vi "resize_table_columns.vi"(7 "vi_reference":refnum<vi>, 8 "error in (no error)":errorcluster, 10 "configuration":T1=enum."all", 11 "listbox_reference":refnum<vi>) -> (0 "error out":errorcluster)   [LabVIEW 2015, in "lv-pagination.lvlib"]
doc: "This VI can be used to automatically determine the appropriate value for column width and row height depending on the contents of the cells themselves."
uses:
  lv-pagination.lvlib
  _controls/configuratin_resize.ctl
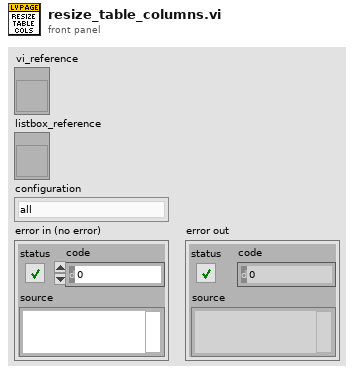
[diagram p1: front panel]
types:
  T1 = typedef "lv-pagination.lvlib/configuratin_resize.ctl" = enum16{"<resize_config>", "header", "contents", "all", "best_fit"}
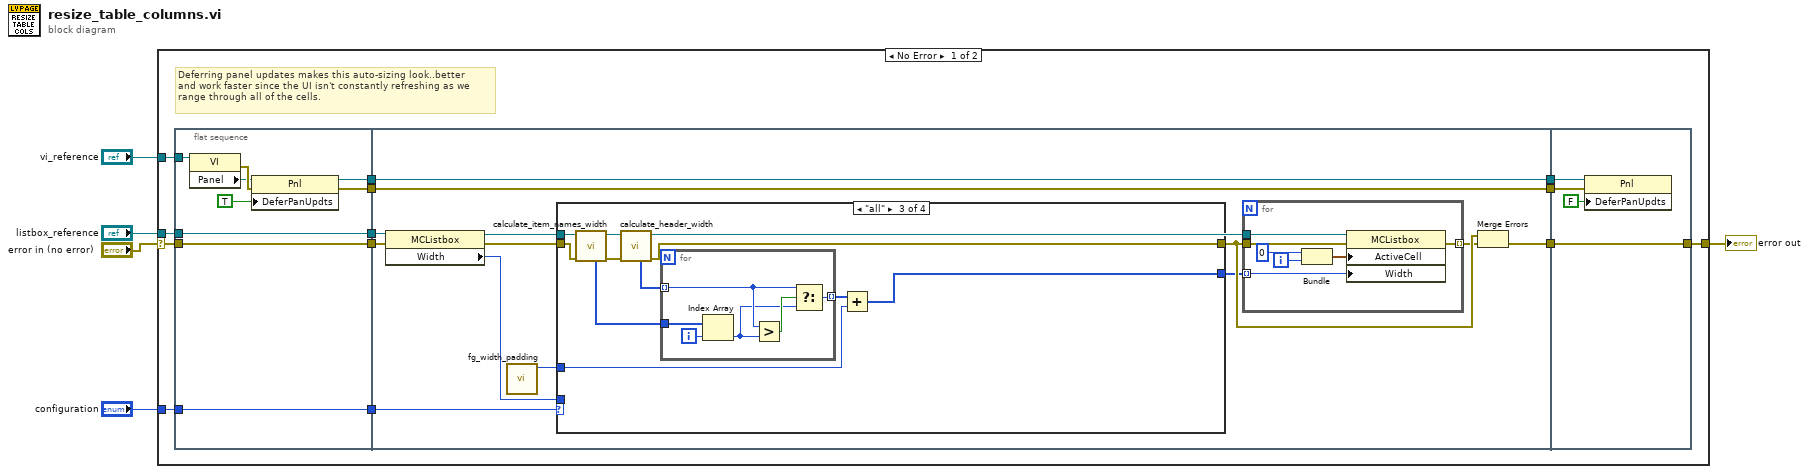
[diagram p0: block diagram]
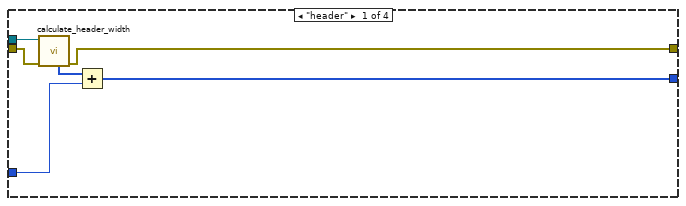
[diagram p2: hidden frame]
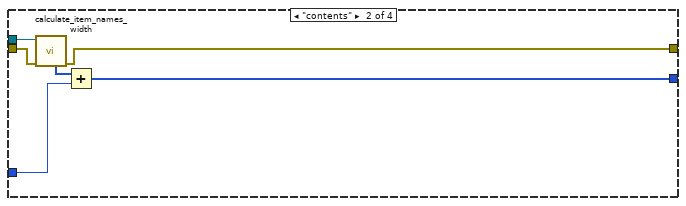
[diagram p3: hidden frame]
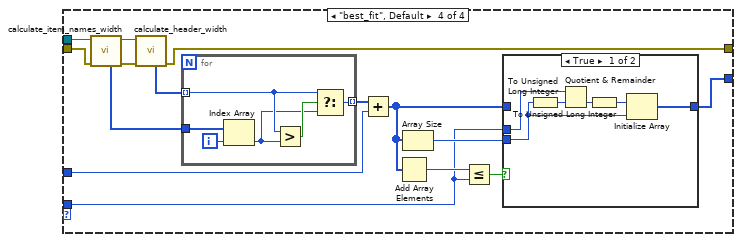
[diagram p4: hidden frame]
diagram:
  n1 = case shown="No Error" "error in (no error)" {
    selector: "error in (no error)" -> [w6 w106]
    tunnel: "configuration" -> [w10 _]
    tunnel: "listbox_reference" -> [w9 _]
    tunnel: [w8 w106] -> w3
    tunnel: "vi_reference" -> [w7 _]
    frame No Error {
      # "Deferring panel updates makes this auto-sizing look..better\nand work faster since the UI isn't constantly refreshing as we\nrange through all of the cells."
      n2 = flat-sequence {
        tunnel: w9 -> [w26]
        tunnel: w10 -> [w27]
        tunnel: [w27] -> w18
        tunnel: [w26] -> w17
        tunnel: w7 -> [w22]
        tunnel: [w21] -> w16
        tunnel: [w20] -> w15
        tunnel: [w19] -> w14
        tunnel: w6 -> [w19]
        tunnel: w18 -> [w40]
        tunnel: w17 -> [w39]
        tunnel: [w38] -> w13
        tunnel: w16 -> [w29]
        tunnel: w15 -> [w30]
        tunnel: [w30] -> w12
        tunnel: [w29] -> w11
        tunnel: w14 -> [w28]
        tunnel: [w105] -> w8
        tunnel: w13 -> [w105]
        tunnel: w12 -> [w104]
        tunnel: w11 -> [w103]
        frame #0 {
          n3 = property class="VI"(reference=w22) -> (error out=w25:errorcluster, "Panel"=w23:refnum<vi>)  [unwired: 1 in, 1 out]
          n4 = property class="Pnl"(reference=w23, error in=w25, "DeferPanUpdts"=TRUE) -> (reference out=w20:refnum<vi>, error out=w21:errorcluster)
        }
        frame #1 {
          n5 = property on="Property Node" class="MCListbox"(reference=w39, error in=w28) -> (reference out=w32:refnum<vi>, error out=w34:errorcluster, "Width"=w33:u32)
          n6 = call "fg_width_padding.vi"() -> ("width_padding out"=w31:u32)  [unwired: 10 in, 1 out]
          n7 = case shown="\"all\"" w40 {
            tunnel: [w46 w51 w55 w71] -> w35
            tunnel: w33 -> [_ _ _ w69]
            tunnel: w31 -> [w45 w52 w56 w76]
            tunnel: w32 -> [w44 w50 w53 w68]
            tunnel: w34 -> [w43 w49 w61 w81]
            tunnel: [w41 w47 w54 w75] -> w37
            frame "header" {
              n8 = call "calculate_header_width.vi"("error in (no error)"=w43, "listbox_reference"=w44) -> ("error out"=w41:errorcluster, "width []"=w42:u32[])  [unwired: 7 in, 1 out]
              n9 = Add(x=w42, y=w45) -> (x+y=w46:u32[])
            }
            frame "contents" {
              n10 = call "calculate_item_names_width.vi"("error in (no error)"=w49, "listbox_reference"=w50) -> ("error out"=w47:errorcluster, "width []"=w48:u32[])  [unwired: 7 in, 1 out]
              n11 = Add(x=w48, y=w52) -> (x+y=w51:u32[])
            }
            frame "all" {
              n12 = call "calculate_item_names_width.vi"("error in (no error)"=w61, "listbox_reference"=w53) -> ("error out"=w60:errorcluster, "width []"=w58:u32[])  [unwired: 7 in, 1 out]
              n13 = call "calculate_header_width.vi"("error in (no error)"=w60, "listbox_reference"=w53) -> ("error out"=w54:errorcluster, "width []"=w59:u32[])  [unwired: 7 in, 1 out]
              n14 = for {
                tunnel: w59 -> [w64] mode=indexing
                tunnel: w58 -> [w67]
                tunnel: [w62] -> w57 mode=indexing
                i -> [w66]
                n15 = Index Array(array=w67, index=w66) -> (element=w63:u32)
                n16 = Greater?(x=w64, y=w63) -> (0:w65:bool)
                n17 = Select(t=w64, s=w65, f=w63) -> (s? t:f=w62:u32)
              }
              n18 = Add(x=w57, y=w56) -> (x+y=w55:u32[])
            }
            frame "best_fit", Default {
              n19 = call "calculate_item_names_width.vi"("error in (no error)"=w81, "listbox_reference"=w68) -> ("error out"=w80:errorcluster, "width []"=w78:u32[])  [unwired: 7 in, 1 out]
              n20 = call "calculate_header_width.vi"("error in (no error)"=w80, "listbox_reference"=w68) -> ("error out"=w75:errorcluster, "width []"=w79:u32[])  [unwired: 7 in, 1 out]
              n21 = for {
                tunnel: w79 -> [w84] mode=indexing
                tunnel: w78 -> [w87]
                tunnel: [w82] -> w77 mode=indexing
                i -> [w86]
                n22 = Index Array(array=w87, index=w86) -> (element=w83:u32)
                n23 = Greater?(x=w84, y=w83) -> (0:w85:bool)
                n24 = Select(t=w84, s=w85, f=w83) -> (s? t:f=w82:u32)
              }
              n25 = Add(x=w77, y=w76) -> (x+y=w70:u32[])
              n26 = Add Array Elements(numeric array=w70) -> (sum=w74:u32)
              n27 = Array Size(array=w70) -> (size(s)=w72:i32)
              n28 = Less Or Equal?(x=w74, y=w69) -> (x <= y?=w73:bool)
              n29 = case shown="True" w73 {
                tunnel: w70 -> [_ w94]
                tunnel: [w93 w94] -> w71
                tunnel: w69 -> [w92 _]
                tunnel: w72 -> [w91 _]
                frame True {
                  n30 = To Unsigned Long Integer(number=w91) -> (unsigned 32bit integer=w88:u32)
                  n31 = Quotient & Remainder(x=w92, y=w88) -> (floor(x/y)=w90:u32)  [unwired: 1 out]
                  n32 = To Unsigned Long Integer(number=w90) -> (unsigned 32bit integer=w89:u32)
                  n33 = Initialize Array(w89, w91) -> (w93:u32[])
                }
                frame False {
                }
              }
            }
          }
          n34 = for {
            tunnel: w32 -> [w101]
            tunnel: [w100] -> w36 mode=indexing
            tunnel: w35 -> [w96] mode=indexing
            tunnel: w37 -> [w95]
            i -> [w98]
            n35 = Bundle("Column"=0, w98) -> (w99:cluster{"Column":i32, i32})  [unwired: 1 in]
            n36 = property on="Property Node" class="MCListbox"(reference=w101, error in=w95, "ActiveCell"=w99, "Width"=w96) -> (error out=w100:errorcluster)  [unwired: 1 out]
          }
          n37 = Merge Errors(w37, w36) -> (w38:errorcluster)
        }
        frame #2 {
          n38 = property class="Pnl"(reference=w104, error in=w103, "DeferPanUpdts"=FALSE ("Defer Panel Updates")) -> ()  [unwired: 2 out]
        }
      }
    }
    frame Error {
    }
  }
  "error out" <- w3
